vi "Read Text File.vi"(8 "error in (no error)":errorcluster, 11 "Path":path) -> (0 "error out":errorcluster, 2 "Data":dbl[](array[numeric]))   [LabVIEW 2022 SP3]
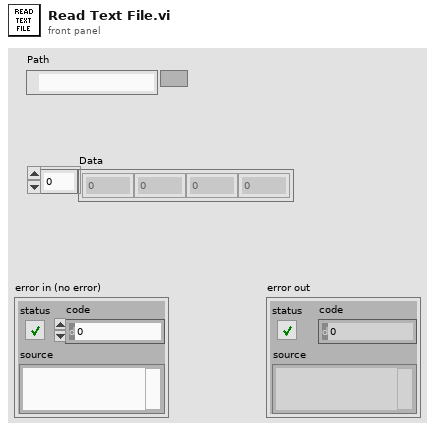
[diagram p1: front panel]
types:
  T1 = enum16{"open", "replace", "create", "open or create", "replace or create", "replace or create with confirmation"}
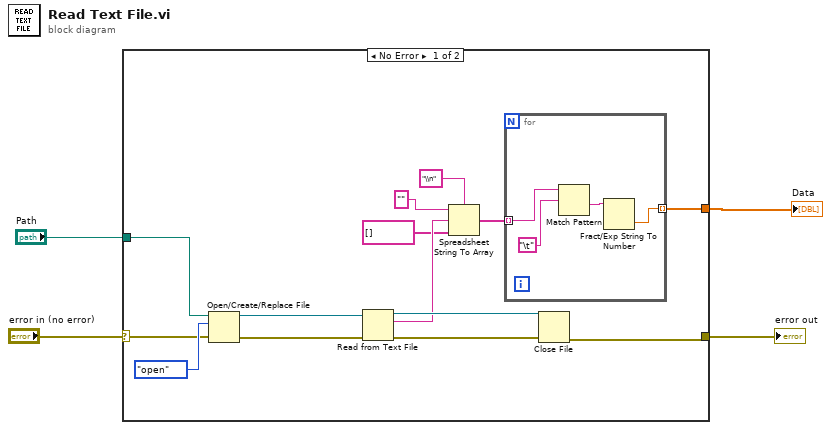
[diagram p0: block diagram]
diagram:
  n1 = case shown="No Error" "error in (no error)" {
    selector: "error in (no error)" -> [w17 w23]
    tunnel: [w15 w23] -> w3
    tunnel: "Path" -> [w16 _]
    tunnel: [w5 _] -> w1
    frame No Error {
      n2 = Open/Create/Replace File(file path (use dialog)=w16, error in=w17, operation (0:open)=T1."open") -> (refnum out=w12:refnum<file>, error out=w14:errorcluster)  [unwired: 3 in, 1 out]
      n3 = Read from Text File(file (use dialog)=w12, error in=w14) -> (refnum out=w11:refnum<file>, text=w10:string, error out=w13:errorcluster)  [unwired: 2 in, 1 out]
      n4 = Spreadsheet String To Array(delimiter (Tab)="\\n", format string="", spreadsheet string=w10, array type (2D Dbl)=string[] []) -> (array=w6:string[])
      n5 = for {
        tunnel: w6 -> [w22] mode=indexing
        tunnel: [w20] -> w5 mode=indexing
        n6 = Match Pattern(string=w22, regular expression="\t") -> (after substring=w19:string)  [unwired: 1 in, 3 out]
        n7 = Fract/Exp String To Number(string=w19) -> (number=w20:dbl)  [unwired: 3 in, 1 out]
      }
      n8 = Close File(refnum=w11, error in=w13) -> (error out=w15:errorcluster)  [unwired: 1 out]
    }
    frame Error {
    }
  }
  "error out" <- w3
  "Data" <- w1
